vi "Execute.vi"(6 "Index [-1]":i32=-1, 7 "Composite Object":refnum<class "CConfig Object.lvclass">, 8 "error in (no error)":errorcluster, 9 "Results":string[][](array[string]), 11 "Config Query in":refnum<class "Delete Query.lvclass">) -> (0 "error out":errorcluster, 1 "Results":string[][](array[string]), 2 "Result":bool, 3 "Config Query out":refnum<class "Delete Query.lvclass">, 4 "Index":i32, 5 "Composite Object":refnum<class "CConfig Object.lvclass">)   [LabVIEW 2013, in "Delete Query.lvclass"]
doc: "Copyright 2018, Carya Automatisering, Wiebe Walstra."
uses:
  Delete Query.lvclass
  CConfig Object.lvclass
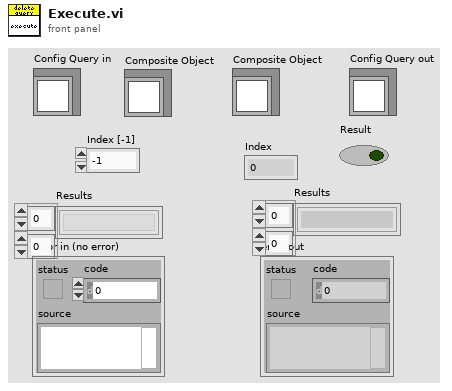
[diagram p1: front panel]
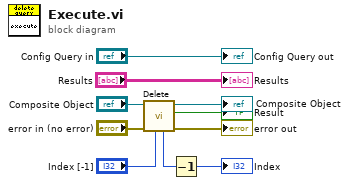
[diagram p0: block diagram]
diagram:
  n1 = call-dynamic "Delete.vi"("Index in"="Index [-1]", "error in (no error)"="error in (no error)", "Composite Object in"="Composite Object") -> ("error out"=→"error out":errorcluster, "Deleted?"=→"Result":bool, "Composite Object out"=→"Composite Object":refnum<class "CConfig Object.lvclass">, "Index in"=w4:i32)  [unwired: 5 in]
  n2 = Decrement(x=w4) -> (x-1=→"Index":i32)
  "Config Query out" <- "Config Query in"
  "Results" <- "Results"
